vi "Output Pulse Train.vi"() -> ()   [LabVIEW 2017]
uses:
  <vilib>/Platform/TimedLoop/XDataNode/timing_clust.ctl
  <vilib>/Platform/TimedLoop/XDataNode/nitl_modes.ctl
  <vilib>/Platform/TimedLoop/XDataNode/wakeup.ctl
  <vilib>/rvi/Emulation/niFpgaGetClockAttributes.vi
  <vilib>/rvi/Emulation/niFpgaSctlEmulationGetInTimedLoop.vi
  <vilib>/rvi/Emulation/niFpgaEmulationReportErrorSimple.vi
  <vilib>/rvi/Emulation/niFpgaCriticalErrorInLSC.vi
  <vilib>/rvi/eio/common/nirviEmuTemplateMethod_errors.vi
  <vilib>/Platform/TimedLoop/XDataNode/XDataNode.xnode
  <vilib>/eio/EIONode/EIONode.xnode
  <vilib>/Platform/TimedLoop/XDataNode/XDNodeRunTimeDep.lvlib
panel:
  in  "u":u32[](array[numeric])=[0, 0, 0, 0, 0, 0, 0, 0, 0, 0, 0, 0, 0, 0, 0, 0, 0, 0, 0, 0, 0, 0, 0, 0, 0, 0, 0, 0, 0, 0, 0, 0, 0, 0, 0, 0, 0, 0, 0, 0, 0, 0, 0, 0, 0, 0, 0, 0, 0, 0, 0, 0, 0, 0, 0, 0, 0, 0, 0, 0, 0, 0, 0, 0, 0, 0, 0, 0, 0, 0, 0, 0, 0, 0, 0, 0, 0, 0, 0, 0, 0, 0, 0, 0, 0, 0, 0, 0, 0, 0, 0, 0, 0, 0, 0, 0, 0, 0, 0, 0, 0, 0, 0, 0, 0, 0, 0, 0, 0, 0, 0, 0, 0, 0, 0, 0, 0, 0, 0, 0, 0, 0, 0, 0, 0, 0, 0, 0, 0, 0, 0, 0, 0, 0, 0, 0, 0, 0, 0, 0, 0, 0, 0, 0, 0, 0, 0, 0, 0, 0, 0, 0, 0, 0, 0, 0, 0, 0, 0, 0, 0, 0, 0, 0, 0, 0, 0, 0, 0, 0, 0, 0, 0, 0, 0, 0, 0, 0, 0, 0, 0, 0, 0, 0, 0, 0, 0, 0, 0, 0, 0, 0, 0, 0, 0, 0, 0, 0, 0, 0, 0]
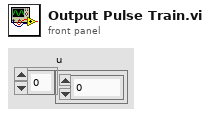
[diagram p1: front panel]
types:
  T1 = typedef "XDNodeRunTimeDep.lvlib/timing_clust.ctl" = cluster{"Expected End [f-1]":u64, "Actual End [f-1]":u64, "Finished Late? [f-1]":bool, "Expected End [i-1]":u64, "Actual End [i-1]":u64, "Finished Late? [i-1]":bool, "Expected Start [i]":u64, "Actual Start [i]":u64, "Expected Start [f]":u64, "Actual Start [f]":u64, "Source Name":string, "Structure Name":string, "Period":i64, "Deadline":i64, "Offset":i64, "Start":i64, "Priority":i32, "Timeout":i32, "Mode":T2, "Wakeup Reason":T3, "Error":errorcluster, "Source Type":string, "Secondary Source Type":string, "Global End Time":u64, "Global Start Time":u64, "Frame Duration":u64, "Iteration Duration":u64, "Assigned CPU":i32, "I/O Scan Engine Mode":u32}
  T2 = typedef "XDNodeRunTimeDep.lvlib/nitl_modes.ctl" = enum32{"No Change", "Process missed periods, maintain original phase", "Discard missed periods, maintain original phase", "Process missed periods, ignore original phase", "Discard missed periods, ignore original phase"}
  T3 = typedef "XDNodeRunTimeDep.lvlib/wakeup.ctl" = enum32{"Normal", "Aborted", "Asynchronous wakeup", "Timing source error", "Timed loop error", "Timeout"}
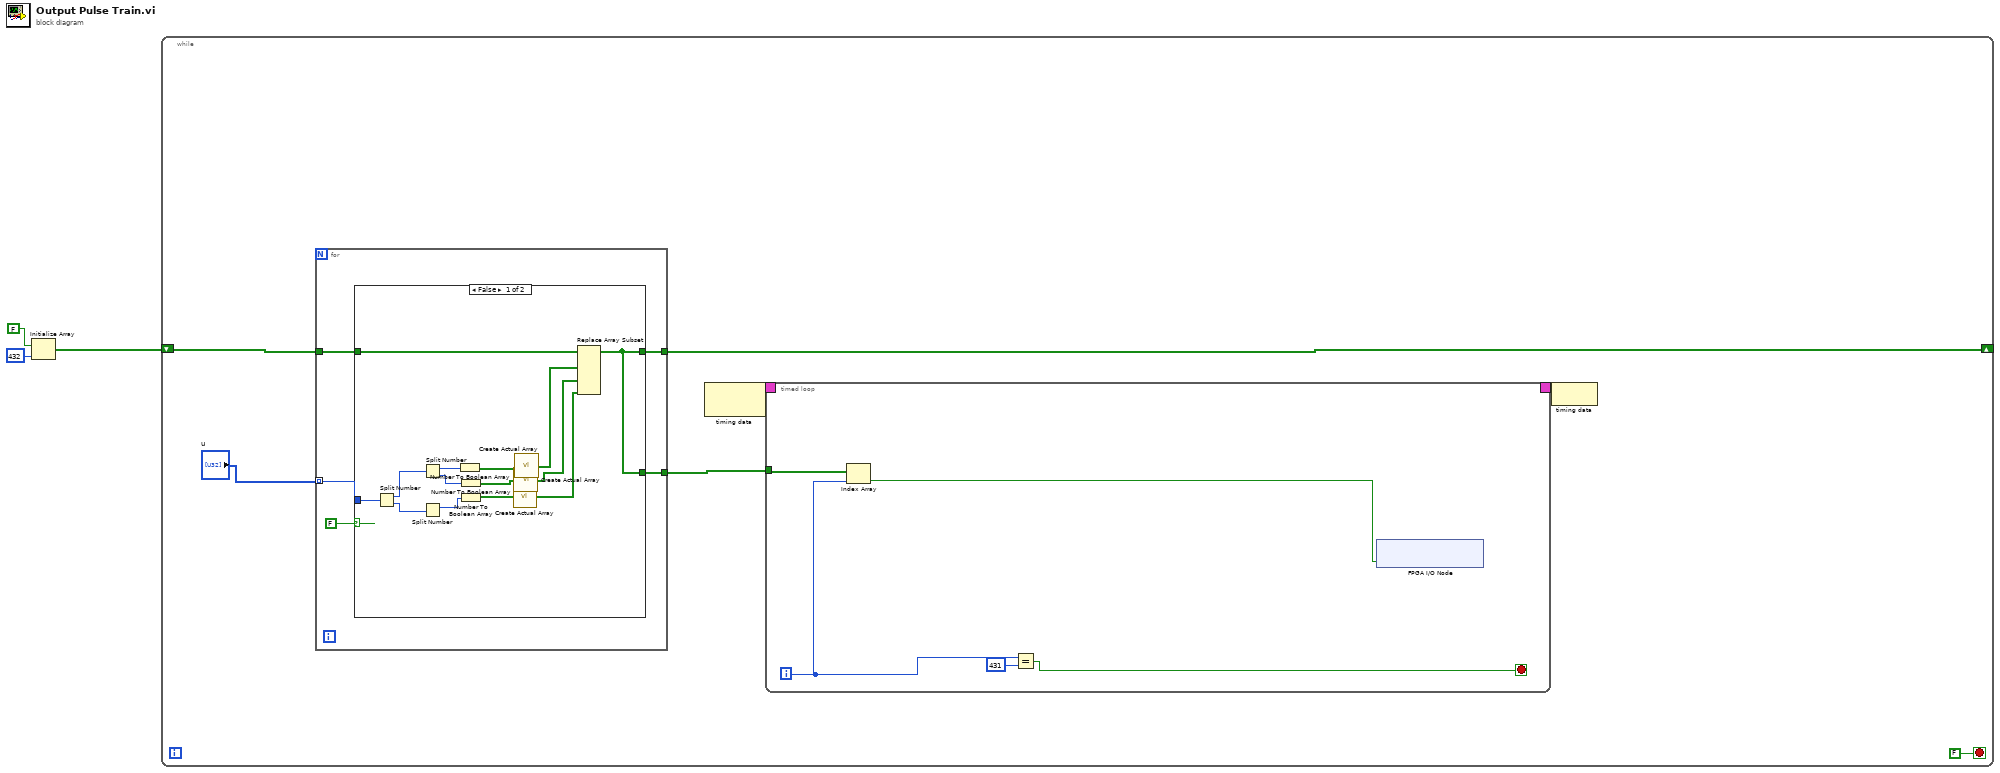
[diagram p0: block diagram]
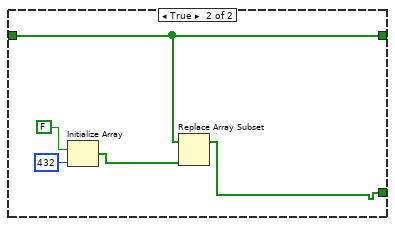
[diagram p2: hidden frame]
diagram:
  n1 = Initialize Array(FALSE, 432 ("dimension size")) -> (w1:bool[])
  n2 = while {
    shift-right: [w5] -> _
    shift-left: w1 -> [w6]
    stop <- FALSE stop-if-true
    n3 = for {
      tunnel: [w15] -> w8
      tunnel: w6 -> [w14]
      tunnel: [w13] -> w5
      tunnel: "u" -> [w11] mode=indexing
      n4 = case shown="False" FALSE {
        tunnel: w11 -> [w16 _]
        tunnel: [w17 w30] -> w15
        tunnel: w14 -> [w21 w31]
        tunnel: [w17 w31] -> w13
        frame False {
          n5 = Split Number(x=w16) -> (hi(x)=w29:u16, lo(x)=w28:u16)
          n6 = Split Number(x=w29) -> (hi(x)=w27:u8, lo(x)=w26:u8)
          n7 = Split Number(x=w28) -> (hi(x)=w25:u8)  [unwired: 1 out]
          n8 = Number To Boolean Array(number=w27) -> (Boolean array=w24:bool[])
          n9 = Number To Boolean Array(number=w26) -> (Boolean array=w23:bool[])
          n10 = Number To Boolean Array(number=w25) -> (Boolean array=w22:bool[])
          n11 = call "Create Actual Array.vi"("Boolean array"=w22) -> ("Ouptut Array"=w18:bool[])
          n12 = call "Create Actual Array.vi"("Boolean array"=w23) -> ("Ouptut Array"=w19:bool[])
          n13 = call "Create Actual Array.vi"("Boolean array"=w24) -> ("Ouptut Array"=w20:bool[])
          n14 = Replace Array Subset(array=w21, new element #1=w20, new element #2=w19, new element #3=w18) -> (w17:bool[])  [unwired: 3 in]
        }
        frame True {
          n15 = Initialize Array(FALSE, 432 ("dimension size")) -> (w32:bool[])
          n16 = Replace Array Subset(array=w31, new element=w32) -> (w30:bool[])  [unwired: 1 in]
        }
      }
    }
    n17 = node-c288() -> (w10:T1)  [unwired: 1 in]
    n18 = timed-loop {
      timing: w10 -> [_]
      timing-out: [_] -> w9
      tunnel: w8 -> [w37]
      i -> [w36]
      stop <- w38 stop-if-true
      n19 = Index Array(array=w37, index=w36) -> (element=w35:bool)
      n20 = Equal?(x=w36, y=431) -> (x = y?=w38:bool)
      n21 = xnode "FPGA I/O Node"("ConnectorC/DIO0"=w35) -> ()  [unwired: 1 in, 1 out]
    }
    n22 = node-c288(w9) -> ()
  }
